vi "iRobot Example - Sensor Stream.vi"() -> ()   [LabVIEW 2014]
doc: "Simplest example for streaming iRobot sensors."
uses:
  Sensor/Bumps + Wheel Drops.ctl
  Sensor/Low-Side Driver + Wheel Overcurrent.ctl
  Sensor/Charging State.ctl
  Sensor/Cargo Bay Digital Inputs.ctl
  Sensor/Charging Sources Available.ctl
  Sensor/Buttons.ctl
  Sensor/OI Mode.ctl
  Sensor/Sensor Group 6.ctl
  Advanced/UART/iRobot UART Port Type.ctl
panel:
  in  "UART port in":T1="ASRL1::INSTR"
  in  "stop":bool
  out "sensors":T2={"Bumps + Wheel Drops"={"Wheeldrop Caster"=FALSE, "Wheeldrop Left"=FALSE, "Wheeldrop Right"=FALSE, "Bump Left"=FALSE, "Bump Right"=FALSE}, "Wall"=FALSE, "Cliff Left"=FALSE, "Cliff Front Left"=FALSE, "Cliff Front Right"=FALSE, "Cliff Right"=FALSE, "Wall Signal"=0, "Cliff Left Signal"=0, "Cliff Front Left Signal"=0, "Cliff Front Right Signal"=0, "Cliff Right Signal"=0, "Buttons"={"Advance"=FALSE, "Play"=FALSE}, "Virtual Wall"=FALSE, "# Stream Packets"=0, "Requested Velocity (mm/s)"=0, "Requested Radius (mm)"=0, "Requested Right Wheel Velocity (mm/s)"=0, "Requested Left Wheel Velocity (mm/s)"=0, "Distance (mm)"=0, "Angle (deg)"=0, "Song Playing"=FALSE, "Song Number"=0, "Charging State"=enum."Not Charging", "Voltage (mV)"=0, "Current (mA)"=0, "Battery Temperature (deg C)"=0, "Battery Charge (mAh)"=0, "Battery Capacity (mAh)"=0, "Charging Sources"={"Internal Charger"=FALSE, "Home Base"=FALSE}, "OI Mode"=enum."Off", "Digital Inputs"={"Digital Input 0"=FALSE, "Digital Input 1"=FALSE, "Digital Input 2"=FALSE, "Digital Input 3"=FALSE, "Device Detect"=FALSE}, "Drivers & Wheel Overcurrent"={"Low-Side Driver 0"=FALSE, "Low-Side Driver 1"=FALSE, "Low-Side Driver 2"=FALSE, "Left Wheel"=FALSE, "Right Wheel"=FALSE}, "Analog Signal"=0, "Infrared"=255} {"Infrared" format="%02x"}
  # "Electrical: charging, battery, OI mode"
  # "Sensors: bump, cliff, button, wheel drop, wall, virtual wall"
  # "Motion: distance, angle, requested velocity"
  # "Cargo Bay: I/O, overcurrent, infrared"
  # "Song"
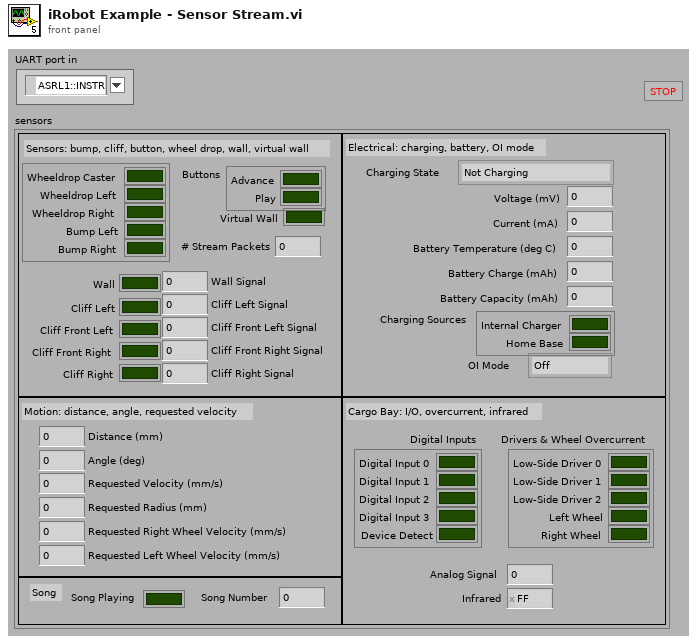
[diagram p1: front panel]
types:
  T1 = typedef "iRobot UART Port Type.ctl" = refnum<visa-resource-name>
  T2 = typedef "Sensor Group 6.ctl" = cluster{"Bumps + Wheel Drops":T3, "Wall":bool, "Cliff Left":bool, "Cliff Front Left":bool, "Cliff Front Right":bool, "Cliff Right":bool, "Wall Signal":u16, "Cliff Left Signal":u16, "Cliff Front Left Signal":u16, "Cliff Front Right Signal":u16, "Cliff Right Signal":u16, "Buttons":T4, "Virtual Wall":bool, "# Stream Packets":u8, "Requested Velocity (mm/s)":i16, "Requested Radius (mm)":i16, "Requested Right Wheel Velocity (mm/s)":i16, "Requested Left Wheel Velocity (mm/s)":i16, "Distance (mm)":i32, "Angle (deg)":i32, "Song Playing":bool, "Song Number":u8, "Charging State":T5, "Voltage (mV)":u16, "Current (mA)":i16, "Battery Temperature (deg C)":i8, "Battery Charge (mAh)":u16, "Battery Capacity (mAh)":u16, "Charging Sources":T6, "OI Mode":T7, "Digital Inputs":T8, "Drivers & Wheel Overcurrent":T9, "Analog Signal":u16, "Infrared":u8}
  T3 = typedef "Bumps + Wheel Drops.ctl" = cluster{"Wheeldrop Caster":bool, "Wheeldrop Left":bool, "Wheeldrop Right":bool, "Bump Left":bool, "Bump Right":bool}
  T4 = typedef "Buttons.ctl" = cluster{"Advance":bool, "Play":bool}
  T5 = typedef "Charging State.ctl" = enum16{"Not Charging", "Reconditioning Charging", "Full Charging", "Trickle Charging", "Waiting", "Charging Fault Condition"}
  T6 = typedef "Charging Sources Available.ctl" = cluster{"Internal Charger":bool, "Home Base":bool}
  T7 = typedef "OI Mode.ctl" = enum16{"Off", "Passive", "Safe", "Full"}
  T8 = typedef "Cargo Bay Digital Inputs.ctl" = cluster{"Digital Input 0":bool, "Digital Input 1":bool, "Digital Input 2":bool, "Digital Input 3":bool, "Device Detect":bool}
  T9 = typedef "Low-Side Driver + Wheel Overcurrent.ctl" = cluster{"Low-Side Driver 0":bool, "Low-Side Driver 1":bool, "Low-Side Driver 2":bool, "Left Wheel":bool, "Right Wheel":bool}
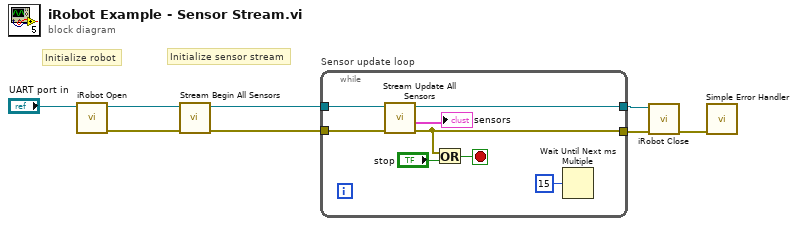
[diagram p0: block diagram]
diagram:
  # "Initialize sensor stream"
  # "Initialize robot"
  n1 = call "iRobot Open.vi"("UART port in"="UART port in") -> ("error out"=w6:errorcluster, "UART port out"=w8:T1)  [unwired: 9 in]
  n2 = call "Stream Begin All Sensors.vi"("error in"=w6, "UART port in"=w8) -> ("error out"=w5:errorcluster, "UART port out"=w7:T1)  [unwired: 8 in]
  n3 = while "Sensor update loop" {
    tunnel: w7 -> [w16]
    tunnel: [w15] -> w3
    tunnel: w5 -> [w13]
    tunnel: [w9] -> w4
    stop <- w11 stop-if-true
    n4 = call "Stream Update All Sensors.vi"("error in"=w13, "UART port in"=w16) -> ("error out"=w9:errorcluster, "sensors"=→"sensors":T2, "UART port out"=w15:T1)  [unwired: 5 in, 2 out]
    n5 = Or(x=w9, y="stop") -> (x .or. y?=w11:bool)
    n6 = Wait Until Next ms Multiple(millisecond multiple=u32 15) -> ()  [unwired: 1 out]
  }
  n7 = call "iRobot Close.vi"("error in"=w4, "UART port in"=w3) -> ("error out"=w2:errorcluster)  [unwired: 9 in]
  n8 = call <vilib>:"Simple Error Handler.vi"("error in (no error)"=w2) -> ()  [unwired: 4 in, 5 out]
